vi "Menu Button - Value Write.vi"(7 "RadioButtonsControl in":refnum<vi>, 9 "Value":string, 10 "Display State In in":T2={"Header"="", "Label[]"=[], "DisableButtonsLUT"=variant(string[] []), "Menu Config"=variant}, 11 "Data In in":T1) -> (2 "Display State In out":T2={"Header"="", "Label[]"=[], "DisableButtonsLUT"=variant(string[] []), "Menu Config"=variant}, 3 "Data In out":T1)   [LabVIEW 2019, in "Menu Button.xctl"]
doc: "JSMA Module Template - Top Level UI 0.2.0.4\nRob Humfeld - Jet Engineering\nCopyright (c) 2019, Jet Engineering"
uses:
  Menu Button.xctl
  State 1.ctl
  Data 1.ctl
  Button Config Cluster STYP.ctl
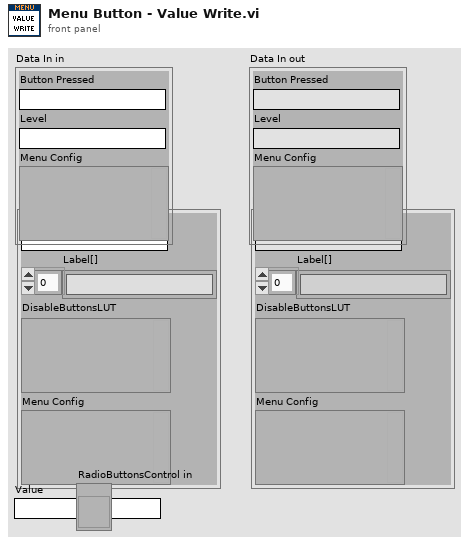
[diagram p1: front panel]
types:
  T1 = typedef "Menu Button.xctl/Data 1.ctl" = cluster{"Button Pressed":string, "Level":string, "Menu Config":variant}
  T2 = typedef "Menu Button.xctl/State 1.ctl" = cluster{"Header":string, "Label[]":string[], "DisableButtonsLUT":variant, "Menu Config":variant}
  T3 = enum32{"No Selection", "System Setup", "System Monitor", "Test Selection", "Data Review", "Radio Selection 5", "Radio Selection 6", "Radio Selection 7", "Radio Selection 8", "Radio Selection 9", "Radio Selection 10"}
  T4 = typedef "Menu Button.xctl/Button Config Cluster STYP.ctl" = cluster{"ID":string, "Name":string, "Action":string, "Value":string, "Enable?":bool, "Color":string}
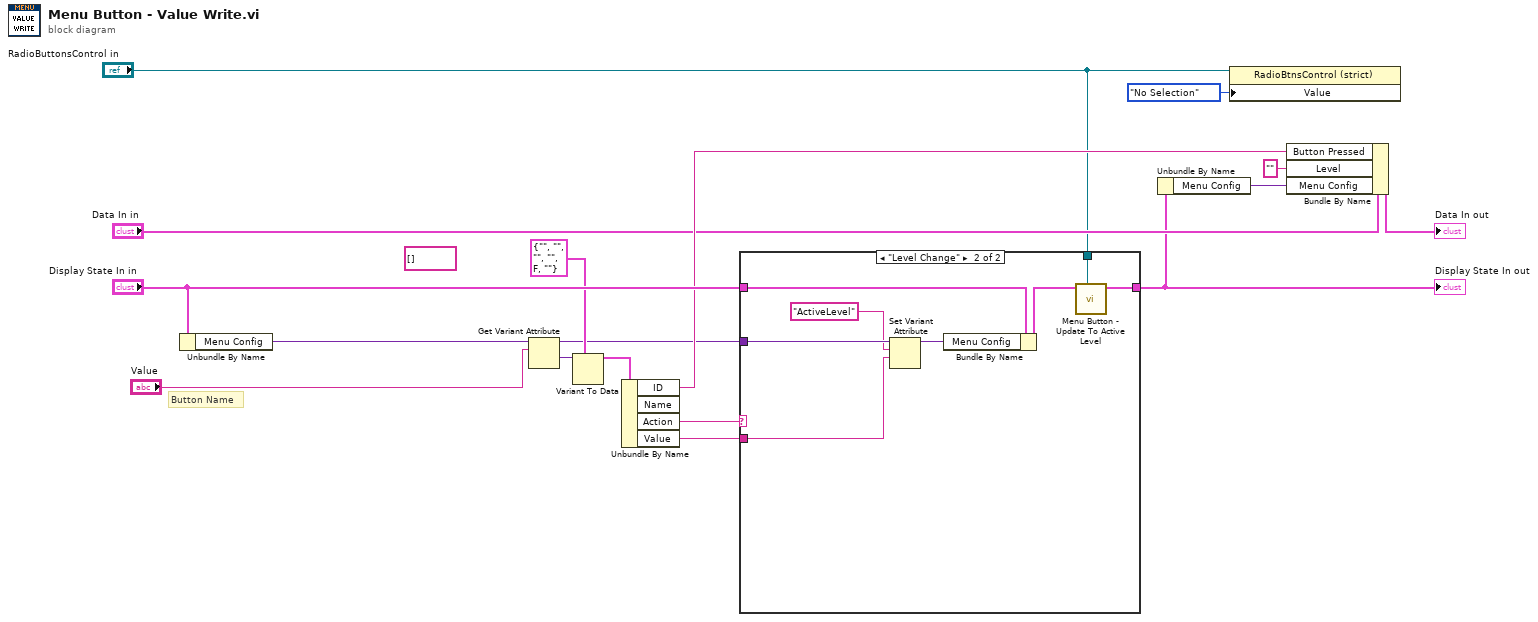
[diagram p0: block diagram]
diagram:
  (unwired) string[] []
  # "Button Name"
  n1 = Unbundle By Name("Display State In in") -> ("Menu Config"=w2:variant)
  n2 = Get Variant Attribute(Variant=w2, name="Value") -> (duplicate Variant=w8:variant, value=w12:variant)  [unwired: 2 in, 2 out]
  n3 = Variant To Data(type=T4 {"ID"="", "Name"="", "Action"="", "Value"="", "Enable?"=FALSE, "Color"=""} ("ButtonConfig"), Variant=w12) -> (data=w9:T4)  [unwired: 1 in, 1 out]
  n4 = Unbundle By Name(w9) -> ("ID"=w15:string, "Action"=w16:string, "Value"=w10:string)  [unwired: 1 out]
  n5 = case shown="\"Level Change\"" w16 {
    tunnel: "Display State In in" -> [w18 w26]
    tunnel: [w18 w23] -> w5
    tunnel: w10 -> [_ w20]
    tunnel: w8 -> [_ w21]
    tunnel: "RadioButtonsControl in" -> [_ w22]
    frame Default {
    }
    frame "Level Change" {
      n6 = Set Variant Attribute(Variant=w21, name="ActiveLevel", value=w20) -> (Variant out=w25:variant)  [unwired: 1 in, 2 out]
      n7 = Bundle By Name(cluster=w26, "Menu Config"=w25) -> (w24:T2)
      n8 = call "Menu Button - Update To Active Level.vi"("RadioButtonsControl in"=w22, "Display State In in"=w24) -> ("Display State In out"=w23:T2)  [unwired: 9 in]
    }
  }
  "Display State In out" <- w5
  n9 = Unbundle By Name(w5) -> ("Menu Config"=w4:variant)
  n10 = property class="RadioBtnsControl (strict)"(reference="RadioButtonsControl in", "Value"=T3."No Selection") -> ()  [unwired: 1 in, 2 out]
  n11 = Bundle By Name(cluster="Data In in", "Button Pressed"=w15, "Level"="", "Menu Config"=w4) -> (→"Data In out":T1)
